vi "Detect.vi"   [LabVIEW 2020, in "feature_detection.lvlib" / "DNN Detection Model.lvclass"]
uses:
  DNN Detection Model.lvclass
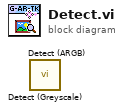
[diagram p0: block diagram]
diagram:
  n1 = call "Detect (Greyscale).vi"() -> ()  [unwired: 9 in, 3 out]
  n2 = call "Detect (ARGB).vi"() -> ()  [unwired: 9 in, 3 out]
